vi "Write Level.vi"(8 "error in (no error)":errorcluster, 10 "Level":T1, 11 "LogRecord in":refnum<class "LogRecord.lvclass">) -> (0 "error out":errorcluster, 3 "LogRecord out":refnum<class "LogRecord.lvclass">)   [LabVIEW 2016, in "hse-logger.lvlib" / "LogRecord.lvclass"]
uses:
  LogRecord.lvclass
  LogLevel.ctl
  LogRecord.lvclass/LogRecord.ctl
  hse-logger.lvlib
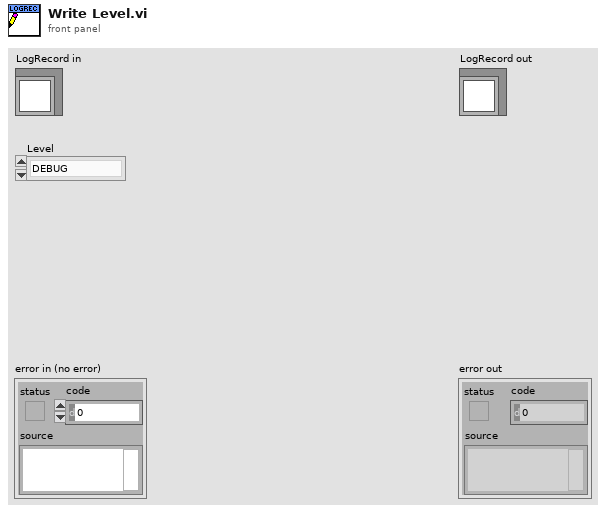
[diagram p1: front panel]
types:
  T1 = typedef "hse-logger.lvlib/LogLevel.ctl" = enum16{"DEBUG", "INFO", "WARNING", "ERROR", "CRITICAL"}
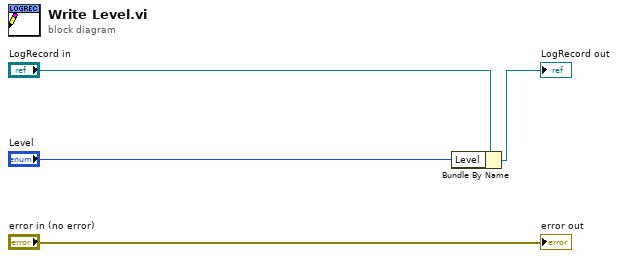
[diagram p0: block diagram]
diagram:
  n1 = Bundle By Name(cluster="LogRecord in", "Level"="Level") -> (→"LogRecord out":refnum<class "LogRecord.lvclass">)
  "error out" <- "error in (no error)"
